vi "Broadcast Single Message.vi"(8 "error in (no error)":errorcluster, 9 "Mail Strategy In":refnum<class "Mail Strategy.lvclass">, 10 "Message In":refnum<class "Message.lvclass">, 11 "Simple Map Queue Group Messenger in":refnum<class "Simple Map Queue Group Messenger.lvclass">) -> (0 "error out":errorcluster, 3 "Simple Map Queue Group Messenger out":refnum<class "Simple Map Queue Group Messenger.lvclass">)   [LabVIEW 2024, in "Simple Map Queue Group Messenger.lvclass"]
uses:
  Simple Map Queue Group Messenger.lvclass
  Ancestor Class/Message/Message.lvclass
  Ancestor Class/Messenger/Mail Strategy/Mail Strategy.lvclass
  Simple Map Queue Group Messenger.lvclass/Simple Map Queue Group Messenger.ctl
  Ancestor Class/Message/Message.lvclass/Message.ctl
  Ancestor Class/Message/Public Data/Read Message Priority.vi
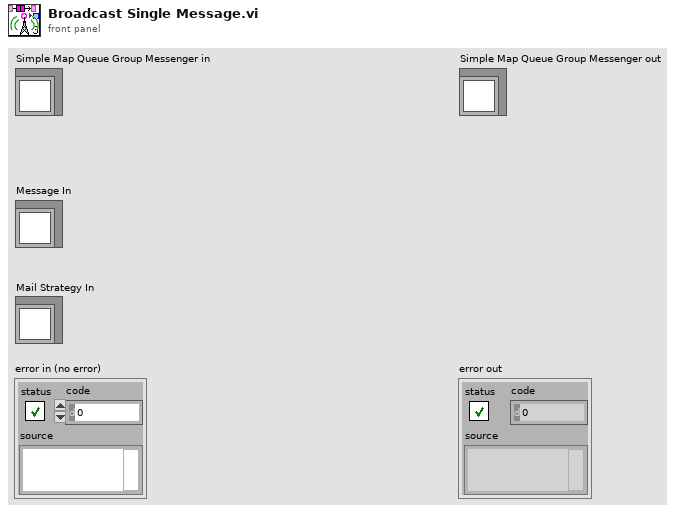
[diagram p1: front panel]
types:
  T1 = typedef "Queue Group Map.ctl" = map{i64, T2[]}
  T2 = typedef "Message Queue.ctl" = refnum<queue>
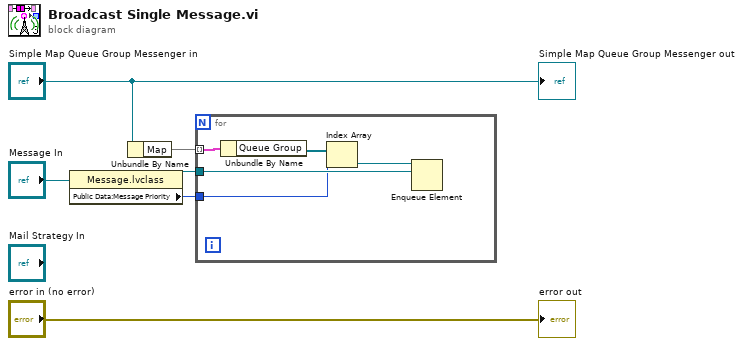
[diagram p0: block diagram]
diagram:
  n1 = property class="Message.lvclass"(reference="Message In") -> (reference out=w2:refnum<class "Message.lvclass">, "Public Data:Message Priority"=w1:i64)  [unwired: 1 in, 1 out]
  n2 = Unbundle By Name("Simple Map Queue Group Messenger in") -> ("Map"=w6:T1)
  n3 = for {
    tunnel: w6 -> [w11] mode=indexing
    tunnel: w2 -> [w8]
    tunnel: w1 -> [w7]
    n4 = Unbundle By Name(w11) -> ("Queue Group"=w10:T2[])
    n5 = Index Array(array=w10, index=w7) -> (element=w9:T2)
    n6 = Enqueue Element(queue=w9, element=w8) -> ()  [unwired: 2 in, 3 out]
  }
  "error out" <- "error in (no error)"
  "Simple Map Queue Group Messenger out" <- "Simple Map Queue Group Messenger in"
